vi "ROI_plot_XY_positions.vi"(0 "Display?":bool, 1 "XYGraph Refnum":refnum<vi>, 2 "XY positions":dbl[][](array[numeric]), 3 "error in":errorcluster, 4 "ROI manager":i32) -> (5 "error out":errorcluster, 6 "XY graph":cluster{dbl[], dbl[]}[](array[cluster]))   [LabVIEW 2015]
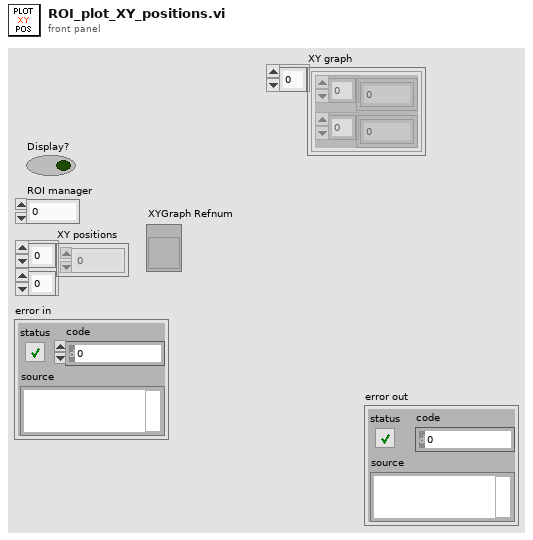
[diagram p1: front panel]
types:
  T1 = typedef "LVRangeTypeDef.ctl" = cluster{"Minimum":dbl, "Maximum":dbl, "Increment":dbl, "Minor Increment":dbl, "Start":dbl}
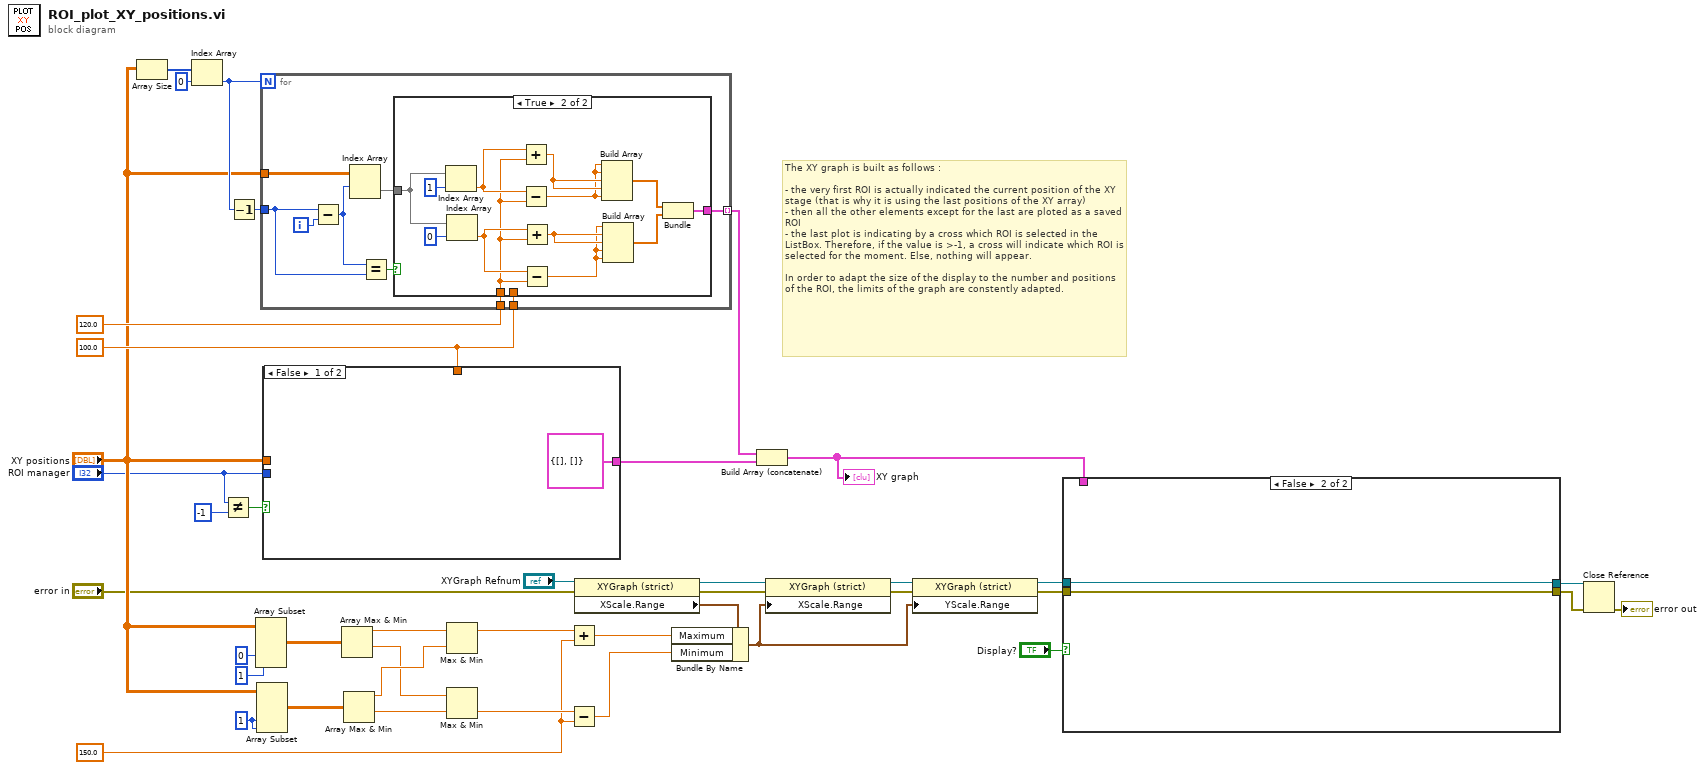
[diagram p0: block diagram]
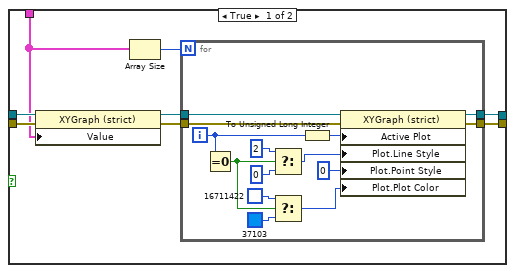
[diagram p2: hidden frame]
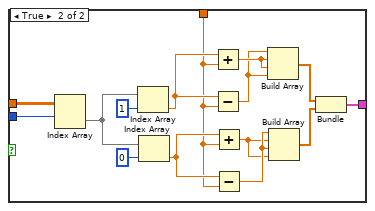
[diagram p3: hidden frame]
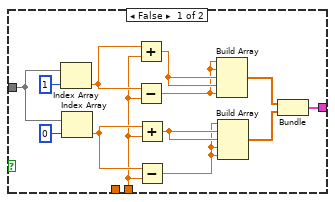
[diagram p4: hidden frame]
diagram:
  w1 = 150.0 ("y")
  w5 = 100.0 ("y")
  w32 = 1 ("index")
  # "The XY graph is built as follows :\n\n- the very first ROI is actually indicated the current position of the XY stage (that is why it is using the last positions of the XY array)\n- then all the other elements except for the last are ploted as a saved ROI\n- the last plot is indicating by a cross which ROI is selected in the ListBox. Therefore, if the value is >-1, a cross will indicate which ROI is selected for the moment. Else, nothing will appear.\n\nIn order to adapt the size of the display to the number and positions of the ROI, the limits of the graph are constently adapted."
  n1 = Array Size(array="XY positions") -> (size(s)=w41:i32[])
  n2 = Index Array(array=w41, index=0) -> (element=w17:i32)
  n3 = Not Equal?(x="ROI manager", y=-1) -> (x != y?=w19:bool)
  n4 = Decrement(x=w17) -> (x-1=w16:i32)
  n5 = Array Subset(array="XY positions", index (col)=0 ("index"), length (col)=1 ("length")) -> (w35:dbl[][])  [unwired: 2 in]
  n6 = Array Subset(array="XY positions", index (col)=w32, length (col)=w32) -> (w34:dbl[][])  [unwired: 2 in]
  n7 = for {
    N: w17 -> [_]
    tunnel: "XY positions" -> [w50]
    tunnel: [w48] -> w21 mode=indexing
    tunnel: w16 -> [w44]
    tunnel: 120.0 ("y") -> [w43]
    tunnel: w5 -> [w42]
    i -> [w46]
    n8 = Subtract(x=w44, y=w46) -> (x-y=w45:i32)
    n9 = Index Array(array=w50, index (row)=w45) -> (element=w49:dbl[])  [unwired: 1 in]
    n10 = Equal?(x=w45, y=w44) -> (x = y?=w47:bool)
    n11 = case shown="True" w47 {
      tunnel: w49 -> [w53 w65]
      tunnel: [w52 w66] -> w48
      tunnel: w43 -> [_ w64]
      tunnel: w42 -> [w51 _]
      frame False {
        n12 = Index Array(array=w53, index=1 ("index (row)")) -> (element=w61:dbl)
        n13 = Index Array(array=w53, index=0 ("index (row)")) -> (element=w58:dbl)
        n14 = Add(x=w61, y=w51) -> (x+y=w60:dbl)
        n15 = Subtract(x=w61, y=w51) -> (x-y=w59:dbl)
        n16 = Add(x=w58, y=w51) -> (x+y=w57:dbl)
        n17 = Subtract(x=w58, y=w51) -> (x-y=w56:dbl)
        n18 = Build Array(w59, w59, w60, w60, w59) -> (w55:dbl[])
        n19 = Build Array(w56, w57, w57, w56, w56) -> (w54:dbl[])
        n20 = Bundle(w55, w54) -> (w52:cluster{dbl[], dbl[]})  [unwired: 1 in]
      }
      frame True {
        n21 = Index Array(array=w65, index=1 ("index (row)")) -> (element=w74:dbl)
        n22 = Index Array(array=w65, index=0 ("index (row)")) -> (element=w71:dbl)
        n23 = Add(x=w74, y=w64) -> (x+y=w73:dbl)
        n24 = Subtract(x=w74, y=w64) -> (x-y=w72:dbl)
        n25 = Add(x=w71, y=w64) -> (x+y=w70:dbl)
        n26 = Subtract(x=w71, y=w64) -> (x-y=w69:dbl)
        n27 = Build Array(w72, w72, w73, w73, w72) -> (w68:dbl[])
        n28 = Build Array(w69, w70, w70, w69, w69) -> (w67:dbl[])
        n29 = Bundle(w68, w67) -> (w66:cluster{dbl[], dbl[]})  [unwired: 1 in]
      }
    }
  }
  n30 = case shown="False" w19 {
    tunnel: "XY positions" -> [_ w92]
    tunnel: "ROI manager" -> [_ w79]
    tunnel: [cluster{dbl[], dbl[]} {[], []} w91] -> w20
    tunnel: w5 -> [_ w78]
    frame False {
    }
    frame True {
      n31 = Index Array(array=w92, index (row)=w79) -> (element=w88:dbl[])  [unwired: 1 in]
      n32 = Index Array(array=w88, index=1 ("index (row)")) -> (element=w87:dbl)
      n33 = Index Array(array=w88, index=0 ("index (row)")) -> (element=w86:dbl)
      n34 = Add(x=w87, y=w78) -> (x+y=w85:dbl)
      n35 = Subtract(x=w87, y=w78) -> (x-y=w84:dbl)
      n36 = Add(x=w86, y=w78) -> (x+y=w82:dbl)
      n37 = Subtract(x=w86, y=w78) -> (x-y=w83:dbl)
      n38 = Build Array(w84, w85, w85, w84) -> (w81:dbl[])
      n39 = Build Array(w83, w82, w83, w82) -> (w80:dbl[])
      n40 = Bundle(w81, w80) -> (w91:cluster{dbl[], dbl[]})  [unwired: 1 in]
    }
  }
  n41 = Array Max & Min(array=w35) -> (max value=w31:dbl, min value=w28:dbl)  [unwired: 2 out]
  n42 = Array Max & Min(array=w34) -> (max value=w30:dbl, min value=w29:dbl)  [unwired: 2 out]
  n43 = Max & Min(x=w31, y=w30) -> (max(x,y)=w27:dbl)  [unwired: 1 out]
  n44 = Max & Min(x=w28, y=w29) -> (min(x,y)=w25:dbl)  [unwired: 1 out]
  n45 = Add(x=w27, y=w1) -> (x+y=w26:dbl)
  n46 = Subtract(x=w25, y=w1) -> (x-y=w24:dbl)
  n47 = property class="XYGraph (strict)"(reference="XYGraph Refnum", error in="error in") -> (reference out=w15:refnum<vi>, error out=w14:errorcluster, "XScale.Range"=w37:T1)
  n48 = Bundle By Name(cluster=w37, "Maximum"=w26, "Minimum"=w24) -> (w22:T1)
  n49 = Build Array (concatenate)(w21, w20) -> (w11:cluster{dbl[], dbl[]}[])
  "XY graph" <- w11
  n50 = property class="XYGraph (strict)"(reference=w15, error in=w14, "XScale.Range"=w22) -> (reference out=w39:refnum<vi>, error out=w38:errorcluster)
  n51 = property class="XYGraph (strict)"(reference=w39, error in=w38, "YScale.Range"=w22) -> (reference out=w13:refnum<vi>, error out=w12:errorcluster)
  n52 = case shown="False" "Display?" {
    tunnel: w13 -> [w100 w116]
    tunnel: w12 -> [w99 w115]
    tunnel: w11 -> [w96 _]
    tunnel: [w94 w115] -> w8
    tunnel: [w95 w116] -> w9
    frame True {
      n53 = property class="XYGraph (strict)"(reference=w100, error in=w99, "Value"=w96) -> (reference out=w98:refnum<vi>, error out=w97:errorcluster)
      n54 = Array Size(array=w96) -> (size(s)=w93:i32)
      n55 = for {
        N: w93 -> [_]
        tunnel: w98 -> [w114]
        tunnel: w97 -> [w113]
        tunnel: [w111] -> w95
        tunnel: [w110] -> w94
        i -> [w109]
        n56 = Equal To 0?(x=w109) -> (x = 0?=w105:bool)
        n57 = Select(t=u8 2, s=w105, f=u8 0 ("Plot.Plot Color")) -> (s? t:f=w106:u8)
        n58 = Select(t=u32 16711422, s=w105, f=u32 37103) -> (s? t:f=w102:u32)
        n59 = To Unsigned Long Integer(number=w109) -> (unsigned 32bit integer=w112:u32)
        n60 = property class="XYGraph (strict)"(reference=w114, error in=w113, "Active Plot"=w112, "Plot.Line Style"=w106, "Plot.Point Style"=u8 0, "Plot.Plot Color"=w102) -> (reference out=w111:refnum<vi>, error out=w110:errorcluster)
      }
    }
    frame False {
    }
  }
  n61 = Close Reference(reference=w9, error in (no error)=w8) -> (error out=→"error out":errorcluster)
